vi "FTP_file_aktuell.vi"(0 "START_STOP":refnum<vi>, 1 "passftp":string, 3 "remotepath":string, 4 "seconds":u32=30 min=30 max=3600 step=30, 5 "temp.csv midnight2":refnum<vi>, 6 "ftpsite":string, 7 "ref_temp3.csv":refnum<file>, 9 "ref_LOCATOR_User.txt":refnum<file>, 10 "ref_temp.csv":refnum<file>, 11 "ref_LOCATOR_User.csv":refnum<file>, 12 "ref_temp2.csv":refnum<file>, 13 "loginftp":string, 15 "remoteinfopath":string) -> ()   [LabVIEW 2010]
uses:
  <vilib>/Utility/error.llb/DialogType.ctl
  <vilib>/Platform/TimedLoop/XDataNode/XDataNode.xnode
  <vilib>/Platform/TimedLoop/XDataNode/timing_clust.ctl
  <vilib>/Platform/TimedLoop/XDataNode/nitl_modes.ctl
  <vilib>/Platform/TimedLoop/XDataNode/wakeup.ctl
  <vilib>/addons/internet/NI_InternetTK_FTP_VIs.lvlib
  <vilib>/Platform/TimedLoop/XDataNode/XDNodeRunTimeDep.lvlib
panel:
  out "Final_size 2":i32
  out "x+y":i32
  out "String 2":string
  out "EOF?":bool
  out "number of lines (all:-1)":i32=-1
  out "x-y":i32
  out "String":string
  out "Final_size":i32
  out "Initial_size":i32
  out "Number of cicles":i32
  out "length of the string":i32
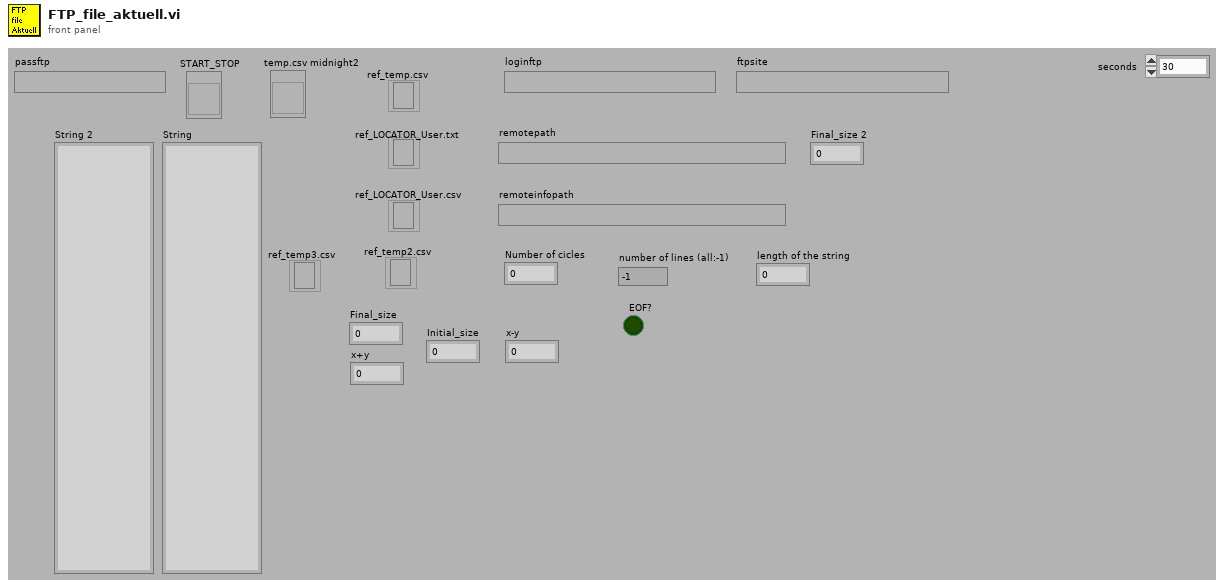
[diagram p1: front panel]
types:
  T1 = typedef "DialogType.ctl" = u16
  T2 = typedef "XDNodeRunTimeDep.lvlib/timing_clust.ctl" = cluster{"Expected End [f-1]":u64, "Actual End [f-1]":u64, "Finished Late? [f-1]":bool, "Expected End [i-1]":u64, "Actual End [i-1]":u64, "Finished Late? [i-1]":bool, "Expected Start [i]":u64, "Actual Start [i]":u64, "Expected Start [f]":u64, "Actual Start [f]":u64, "Source Name":string, "Structure Name":string, "Period":i64, "Deadline":i64, "Offset":i64, "Start":i64, "Priority":i32, "Timeout":i32, "Mode":T3, "Wakeup Reason":T4, "Error":errorcluster, "Source Type":string, "Secondary Source Type":string, "Global End Time":u64, "Global Start Time":u64, "Frame Duration":u64, "Iteration Duration":u64, "Assigned CPU":i32, "I/O Scan Engine Mode":u32}
  T3 = typedef "XDNodeRunTimeDep.lvlib/nitl_modes.ctl" = enum32{"No Change", "Process missed periods, maintain original phase", "Discard missed periods, maintain original phase", "Process missed periods, ignore original phase", "Discard missed periods, ignore original phase"}
  T4 = typedef "XDNodeRunTimeDep.lvlib/wakeup.ctl" = enum32{"Normal", "Aborted", "Asynchronous wakeup", "Timing source error", "Timed loop error", "Timeout"}
  T5 = cluster{"second":i32, "minute":i32, "hour":i32, "day of month":i32, "month":i32, "year":i32, "day of week":i32, "day of year":i32, "is DST":i32}
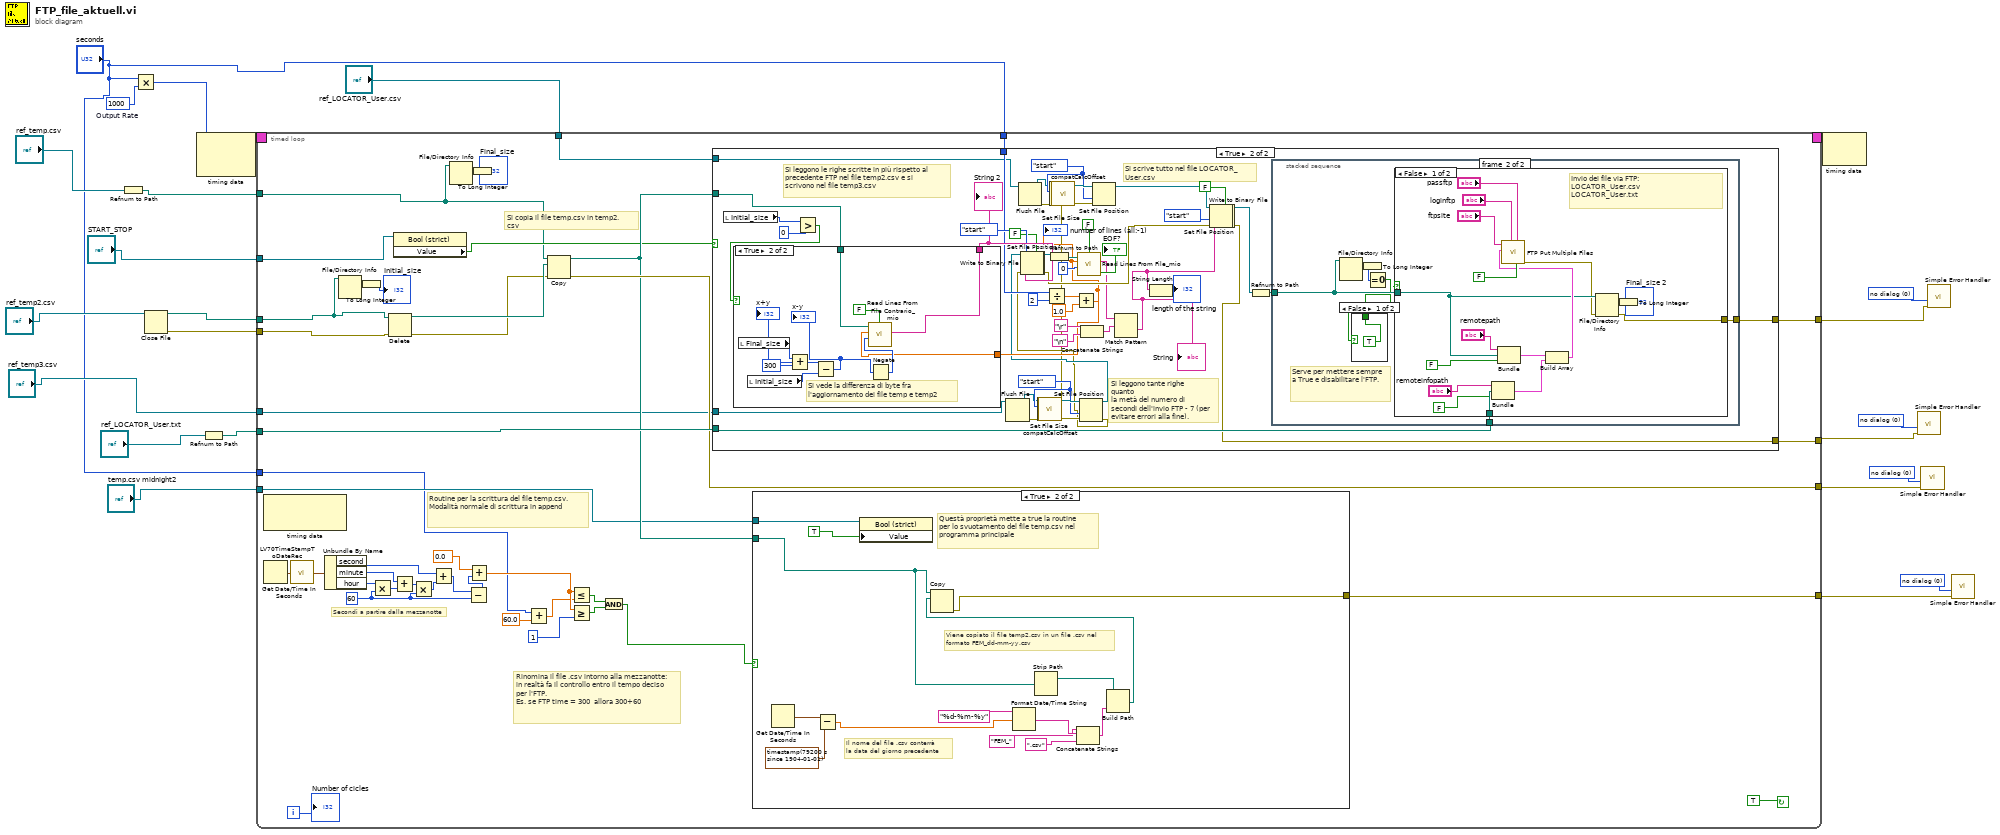
[diagram p0: block diagram]
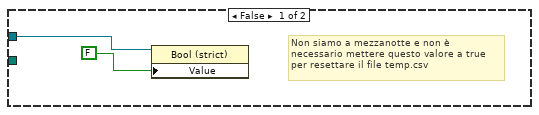
[diagram p2: hidden frame]
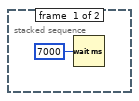
[diagram p4: hidden frame]
diagram:
  w4 = T1 0 items=["no dialog", "OK message", "continue or stop message", "OK message + warnings", "continue/stop + warnings"] ("type of dialog (OK msg:1)")
  w8 = u32 1000  # Output Rate
  w12 = T1 0 items=["no dialog", "OK message", "continue or stop message", "OK message + warnings", "continue/stop + warnings"] ("type of dialog (OK msg:1)")
  w13 = T1 0 items=["no dialog", "OK message", "continue or stop message", "OK message + warnings", "continue/stop + warnings"] ("type of dialog (OK msg:1)")
  w14 = T1 0 items=["no dialog", "OK message", "continue or stop message", "OK message + warnings", "continue/stop + warnings"] ("type of dialog (OK msg:1)")
  n1 = Refnum to Path(1:"ref_temp.csv") -> (0:w21:path)
  n2 = Multiply(x="seconds", y=w8) -> (x*y=w6:u32)
  n3 = Close File(refnum="ref_temp2.csv") -> (path=w20:path, error out=w19:errorcluster)  [unwired: 1 in]
  n4 = node-c288(w6) -> (w1:T2)  [unwired: 1 in]
  n5 = Refnum to Path(1:"ref_LOCATOR_User.txt") -> (0:w23:path)
  n6 = timed-loop {
    tunnel: [w28] -> w3
    tunnel: "seconds" -> [w29]
    tunnel: "ref_temp3.csv" -> [w30]
    tunnel: "seconds" -> [w35]
    timing-out: [_] -> w2
    timing: w1 -> [_]
    tunnel: "temp.csv midnight2" -> [w40]
    tunnel: [w43] -> w11
    tunnel: [w44] -> w15
    tunnel: "ref_LOCATOR_User.csv" -> [w42]
    tunnel: w19 -> [w36]
    tunnel: w20 -> [w34]
    tunnel: [w47] -> w16
    tunnel: w23 -> [w65]
    tunnel: "START_STOP" -> [w66]
    tunnel: w21 -> [w32]
    i -> [w39]
    stop <- TRUE continue-if-true
    w56 = 60
    # "Routine per la scrittura del file temp.csv.\nModalità normale di scrittura in append"
    # "Si copia il file temp.csv in temp2.csv"
    # "Rinomina il file .csv intorno alla mezzanotte:\nin realtà fa il controllo entro il tempo deciso per l'FTP.\nEs. se FTP time = 300  allora 300+60"
    # "Secondi a partire dalla mezzanotte"
    n7 = node-c288() -> ()  [unwired: 1 in, 2 out]
    n8 = Get Date/Time In Seconds() -> (seconds since 1Jan1904=w25:timestamp)
    n9 = call <vilib>:"LV70TimeStampToDateRec.vi"("time stamp"=w25) -> ("date time rec"=w52:T5)
    n10 = Unbundle By Name(w52) -> ("second"=w59:i32, "minute"=w58:i32, "hour"=w53:i32)
    n11 = File/Directory Info(path=w34) -> (size=w26:i64)  [unwired: 1 in, 6 out]
    n12 = To Long Integer(number=w26) -> (32bit integer=→"Initial_size":i32)
    n13 = Multiply(x=w53, y=w56) -> (x*y=w54:i32)
    n14 = Delete(path (use dialog)=w34, error in=w36) -> (deleted path=w38:path, error out=w37:errorcluster)  [unwired: 3 in, 1 out]
    n15 = Add(x=w58, y=w54) -> (x+y=w55:i32)
    n16 = property class="Bool (strict)"(reference=w66) -> ("Value"=w45:bool)  [unwired: 1 in, 2 out]
    n17 = Multiply(x=w55, y=w56) -> (x*y=w57:i32)
    n18 = Add(x=w59, y=w57) -> (x+y=w60:i32)
    n19 = File/Directory Info(path=w32) -> (size=w27:i64)  [unwired: 1 in, 6 out]
    n20 = Subtract(x=w60, y=w56) -> (x-y=w51:i32)
    n21 = Add(x=sgl 0.0, y=w51) -> (x+y=w64:sgl)
    n22 = To Long Integer(number=w27) -> (32bit integer=→"Final_size":i32)
    n23 = Add(x=w35, y=60.0) -> (x+y=w48:dbl)
    n24 = Copy(8:w37, 10:w38, 11:w32) -> (0:w47:errorcluster, 3:w46:path)  [unwired: 2 in, 1 out]
    n25 = Less Or Equal?(x=w64, y=w48) -> (x <= y?=w62:bool)
    n26 = Greater Or Equal?(x=w64, y=1) -> (x >= y?=w61:bool)
    n27 = And(x=w62, y=w61) -> (x .and. y?=w41:bool)
    n28 = case shown="True" w45 {
      tunnel: w46 -> [_ w126]
      tunnel: w65 -> [_ w141]
      tunnel: w42 -> [_ w103]
      tunnel: [_ w100] -> w44
      tunnel: w30 -> [_ w113]
      tunnel: w29 -> [_ w132]
      tunnel: [_ w97] -> w28
      frame False {
      }
      frame True {
        w106 = enum16{"start", "end", "current"}."start" ("pos mode (0:2)")
        w114 = enum16{"start", "end", "current"}."start" ("pos mode (0:2)")
        # "Si scrive tutto nel file LOCATOR_User.csv"
        # "Si leggono tante righe quanto\nla metà del numero di secondi dell'invio FTP - 7 (per evitare errori alla fine)."
        # "Si leggono le righe scritte in più rispetto al precedente FTP nel file temp2.csv e si scrivono nel file temp3.csv"
        n29 = local read "Initial_size"() -> (w136:i32)
        n30 = Greater?(x=w136, y=0) -> (0:w139:bool)
        n31 = Flush File(refnum=w103) -> (refnum out=w105:refnum<file>, error out=w104:errorcluster)  [unwired: 1 in]
        n32 = Divide(x=w132, y=u32 2) -> (x/y=w130:dbl)
        n33 = call <vilib>:"compatCalcOffset.vi"("error in"=w104, "pos mode (0:1)"=w106, "refnum"=w105) -> ("error out"=w96:errorcluster, "offset"=w95:i32, "dup refnum"=w94:refnum<file>)  [unwired: 6 in]
        n34 = Set File Size(4:w96, 6:w95, 7:w94) -> (0:w108:errorcluster, 3:w107:refnum<file>)
        n35 = Add(x=w130, y=1.0) -> (x+y=w117:dbl)
        "number of lines (all:-1)" <- w117
        n36 = case shown="True" w139 {
          tunnel: w126 -> [_ w170]
          tunnel: [_ w176] -> w135
          tunnel: w117 -> [_ w169]
          frame False {
          }
          frame True {
            # "Si vede la differenza di byte fra l'aggiornamento dei file temp e temp2"
            n37 = local read "Final_size"() -> (w172:i32)
            n38 = local read "Initial_size"() -> (w175:i32)
            n39 = Add(x=w172, y=300) -> (x+y=w173:i32)
            "x+y" <- w173
            n40 = Subtract(x=w173, y=w175) -> (x-y=w174:i32)
            "x-y" <- w174
            n41 = Negate(x=w174) -> (-x=w177:i32)
            n42 = call "Read Lines From File Contrario_mio.vi"("convert eol? (no:F)"=FALSE ("line mode (F)"), "file path (dialog if empty)"=w170, "number of lines (all:-1)"=w169, "start of read offset (chars.:0)"=w177) -> ("line string"=w176:string)  [unwired: 2 in, 3 out]
          }
        }
        "String 2" <- w135
        n43 = Concatenate Strings("\r", "\n") -> (w121:string)
        n44 = Set File Position(refnum=w107, from (0:start)=w106, error in=w108) -> (refnum out=w102:refnum<file>, error out=w101:errorcluster)  [unwired: 1 in]
        n45 = Flush File(refnum=w113, error in=w101) -> (refnum out=w112:refnum<file>, error out=w110:errorcluster)
        n46 = call <vilib>:"compatCalcOffset.vi"("error in"=w110, "pos mode (0:1)"=w114, "refnum"=w112) -> ("error out"=w93:errorcluster, "offset"=w92:i32, "dup refnum"=w91:refnum<file>)  [unwired: 6 in]
        n47 = Set File Size(4:w93, 6:w92, 7:w91) -> (0:w116:errorcluster, 3:w115:refnum<file>)
        n48 = Set File Position(refnum=w115, from (0:start)=w114, error in=w116) -> (refnum out=w111:refnum<file>, error out=w109:errorcluster)  [unwired: 1 in]
        n49 = Set File Position(refnum=w111, from (0:start)=enum16{"start", "end", "current"}."start" ("pos mode (0:2)"), error in=w109) -> (refnum out=w90:refnum<file>, error out=w89:errorcluster)  [unwired: 1 in]
        n50 = Write to Binary File(file (use dialog)=w90, data=w135, error in=w89, 5:FALSE ("prepend array or string size? (T)")) -> (refnum out=w133:refnum<file>, error out=w129:errorcluster)  [unwired: 2 in, 1 out]
        n51 = Refnum to Path(1:w133) -> (0:w125:path)
        n52 = call "Read Lines From File_mio.vi"("convert eol? (no:F)"=FALSE, "file path (dialog if empty)"=w125, "number of lines (all:-1)"=w117, "start of read offset (chars.:0)"=0) -> ("line string"=w123:string, "EOF?"=→"EOF?":bool)  [unwired: 2 in, 2 out]
        n53 = Match Pattern(string=w123, regular expression=w121) -> (after substring=w122:string)  [unwired: 1 in, 3 out]
        "String" <- w122
        n54 = String Length(string=w122) -> (length=→"length of the string":i32)
        n55 = Set File Position(refnum=w102, from (0:start)=enum16{"start", "end", "current"}."start" ("pos mode (0:2)"), error in=w129) -> (refnum out=w87:refnum<file>, error out=w86:errorcluster)  [unwired: 1 in]
        n56 = Write to Binary File(file (use dialog)=w87, data=w122, error in=w86, 5:FALSE ("prepend array or string size? (T)")) -> (refnum out=w99:refnum<file>, error out=w100:errorcluster)  [unwired: 2 in, 1 out]
        n57 = Refnum to Path(1:w99) -> (0:w98:path)
        n58 = stacked-sequence {
          tunnel: w141 -> [_ w149]
          tunnel: w98 -> [_ w146]
          tunnel: [_ w148] -> w97
          frame #0 {
            n59 = Wait (ms)(milliseconds to wait=u32 7000) -> ()  [unwired: 1 out]
          }
          frame #1 {
            # "Serve per mettere sempre\na True e disabilitare l'FTP."
            n60 = File/Directory Info(path=w146) -> (size=w145:i64)  [unwired: 1 in, 6 out]
            n61 = To Long Integer(number=w145) -> (32bit integer=w147:i32)
            n62 = Equal To 0?(x=w147) -> (x = 0?=w144:bool)
            n63 = case shown="False" w144 {
              selector: w144 -> [_ w151]
              tunnel: [TRUE w151] -> w143
              frame False {
              }
              frame True {
              }
            }
            n64 = case shown="False" w143 {
              tunnel: w149 -> [w161 _]
              tunnel: w146 -> [w155 _]
              tunnel: [w153 _] -> w148
              frame False {
                # "Invio dei file via FTP:\nLOCATOR_User.csv\nLOCATOR_User.txt"
                n65 = Bundle("remoteinfopath"="remoteinfopath", w161, FALSE) -> (w159:cluster{"remoteinfopath":string, path, bool})  [unwired: 1 in]
                n66 = Bundle("remotepath"="remotepath", w155, FALSE) -> (w157:cluster{"remotepath":string, path, bool})  [unwired: 1 in]
                n67 = Build Array(w157, w159) -> (w158:cluster{"remoteinfopath":string, path, bool}[])
                n68 = call <vilib>:"FTP Put Multiple Files.vi"("active (T)"=FALSE, "password"="passftp", "user"="loginftp", "file specifications"=w158, "host"="ftpsite") -> ("error out"=w154:errorcluster)  [unwired: 5 in, 1 out]
                n69 = File/Directory Info(path=w155, error in=w154) -> (size=w152:i64, error out=w153:errorcluster)  [unwired: 5 out]
                n70 = To Long Integer(number=w152) -> (32bit integer=→"Final_size 2":i32)
              }
              frame True {
                # "Se il file da inviare via FTP è di 0 bytes, non lo inviare."
              }
            }
          }
        }
      }
    }
    n71 = case shown="True" w41 {
      tunnel: w46 -> [_ w77]
      tunnel: [_ w73] -> w43
      tunnel: w40 -> [w70 w71]
      frame False {
        # "Non siamo a mezzanotte e non è necessario mettere questo valore a true per resettare il file temp.csv"
        n72 = property class="Bool (strict)"(reference=w70, "Value"=FALSE) -> ()  [unwired: 1 in, 2 out]
      }
      frame True {
        # "Viene copiato il file temp2.csv in un file .csv nel\nformato FEM_dd-mm-yy.csv"
        # "Il nome del file .csv conterrà\nla data del giorno precedente"
        # "Questà proprietà mette a true la routine per lo svuotamento del file temp.csv nel programma principale"
        n73 = Get Date/Time In Seconds() -> (seconds since 1Jan1904=w76:timestamp)
        n74 = Subtract(x=w76, y=timestamp(79200 s since 1904-01-01)) -> (x-y=w74:dbl)
        n75 = property class="Bool (strict)"(reference=w71, "Value"=TRUE) -> ()  [unwired: 1 in, 2 out]
        n76 = Format Date/Time String(time format string (%c)="%d-%m-%y", seconds (now)=w74) -> (date/time string=w82:string)  [unwired: 1 in]
        n77 = Strip Path(path=w77) -> (stripped path=w79:path)  [unwired: 1 out]
        n78 = Concatenate Strings("FEM_", w82, ".csv") -> (w84:string)
        n79 = Build Path(base path=w79, name or relative path=w84) -> (appended path=w78:path)
        n80 = Copy(10:w78, 11:w77) -> (0:w73:errorcluster)  [unwired: 3 in, 2 out]
      }
    }
    "Number of cicles" <- w39
  }
  n81 = node-c288(w2) -> ()  [unwired: 1 out]
  n82 = call <vilib>:"Simple Error Handler.vi"("type of dialog (OK msg:1)"=w14, "error in (no error)"=w15) -> ()  [unwired: 3 in, 5 out]
  n83 = call <vilib>:"Simple Error Handler.vi"("type of dialog (OK msg:1)"=w13, "error in (no error)"=w16) -> ()  [unwired: 3 in, 5 out]
  n84 = call <vilib>:"Simple Error Handler.vi"("type of dialog (OK msg:1)"=w4, "error in (no error)"=w3) -> ()  [unwired: 3 in, 5 out]
  n85 = call <vilib>:"Simple Error Handler.vi"("type of dialog (OK msg:1)"=w12, "error in (no error)"=w11) -> ()  [unwired: 3 in, 5 out]
